vi "MovingAverage.vi"(2 "Additional Value":dbl, 3 "# to Average":i32) -> (0 "Moving Average":dbl, 1 "Full Set of Values?":bool)   [LabVIEW 2011]
doc: "This stores and averages a moving window of the last n values passed in"
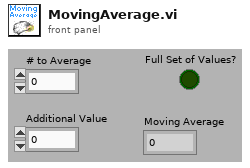
[diagram p1: front panel]
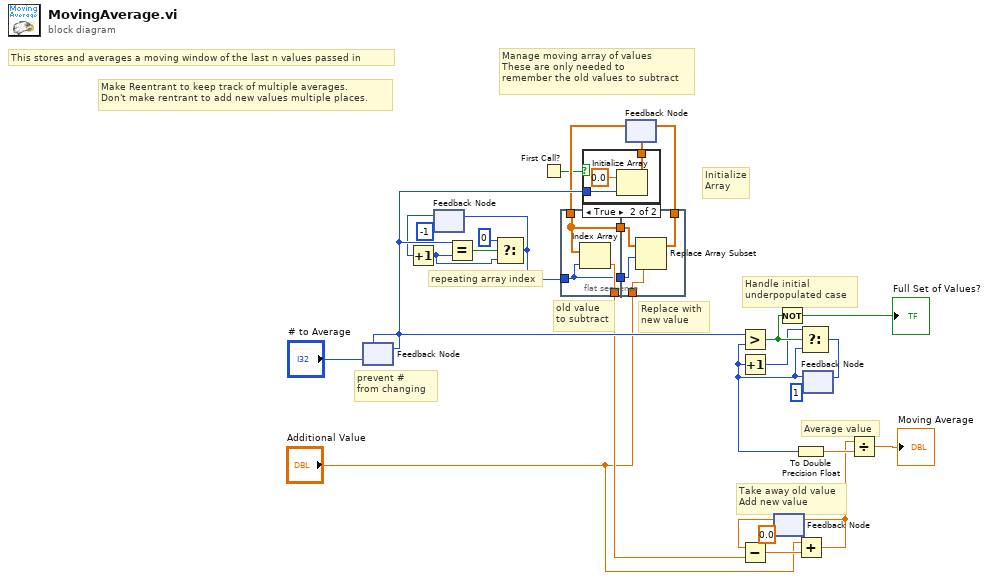
[diagram p0: block diagram]
diagram:
  # "Initialize\nArray"
  # "prevent #\nfrom changing"
  # "This stores and averages a moving window of the last n values passed in"
  # "Make Reentrant to keep track of multiple averages.\nDon't make rentrant to add new values multiple places."
  # "Manage moving array of values\nThese are only needed to \nremember the old values to subtract"
  # "Take away old value\nAdd new value"
  # "Replace with\nnew value"
  # "old value\nto subtract"
  # "Handle initial\nunderpopulated case"
  # "repeating array index"
  # "Average value"
  n1 = feedback #1("# to Average") -> (w20:i32)
  n2 = feedback-in #1(w20) -> ()
  n3 = feedback #2(-1) -> (w15:i32)
  n4 = Increment(x=w15) -> (x+1=w18:i32)
  n5 = Equal?(x=w20, y=w18) -> (x = y?=w16:bool)
  n6 = Select(t=0, s=w16, f=w18) -> (s? t:f=w7:i32)
  n7 = feedback-in #2(w7) -> ()
  n8 = First Call?() -> (First Call?: T/F=w1:bool)
  n9 = flat-sequence {
    tunnel: w8 -> [w30]
    tunnel: w7 -> [w29]
    tunnel: [w31] -> w6
    tunnel: [w30] -> w5
    tunnel: [w29] -> w4
    tunnel: w5 -> [w35]
    tunnel: w4 -> [w34]
    tunnel: "Additional Value" -> [w33]
    tunnel: [w32] -> w2
    frame #0 {
      n10 = Index Array(array=w30, index=w29) -> (element=w31:dbl)
    }
    frame #1 {
      n11 = Replace Array Subset(array=w35, new element=w33, index=w34) -> (w32:dbl[])
    }
  }
  n12 = case shown="True" w1 {
    tunnel: w20 -> [_ w38]
    tunnel: [_ w37] -> w12
    frame False {
    }
    frame True {
      n13 = Initialize Array(0.0 ("Initialize"), w38) -> (w37:dbl[])
    }
  }
  n14 = feedback-in #3(w2) -> ()
  n15 = feedback #3(w12) -> (w8:dbl[])
  n16 = feedback #4(0.0) -> (w27:dbl)
  n17 = Subtract(x=w27, y=w6) -> (x-y=w10:dbl)
  n18 = Add(x="Additional Value", y=w10) -> (x+y=w11:dbl)
  n19 = feedback-in #4(w11) -> ()
  n20 = feedback #5(1) -> (w22:i32)
  n21 = Greater?(x=w20, y=w22) -> (0:w25:bool)
  n22 = Increment(x=w22) -> (x+1=w21:i32)
  n23 = Not(x=w25) -> (.not. x?=→"Full Set of Values?":bool)
  n24 = To Double Precision Float(number=w22) -> (double precision float=w14:dbl)
  n25 = Select(t=w21, s=w25, f=w22) -> (s? t:f=w23:i32)
  n26 = feedback-in #5(w23) -> ()
  n27 = Divide(x=w11, y=w14) -> (x/y=→"Moving Average":dbl)
